vi "svx_Orbit IndexToCheckbox.vi"(4 "All Children Tags":string[](array[string]), 6 "All parents Tags":string[](array[string]), 9 "ColumnIdx":i32, 10 "RowIdx":i32, 11 "Tree ref in":refnum<vi>) -> (3 "Tree ref out":refnum<vi>)   [LabVIEW 2017, in "SVX Orbit.xctl"]
uses:
  <vilib>/addons/_XControls/Orbit Plot/SVX Orbit.xctl
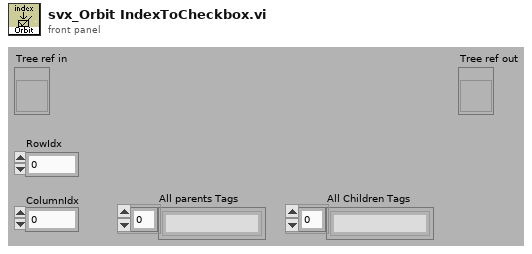
[diagram p1: front panel]
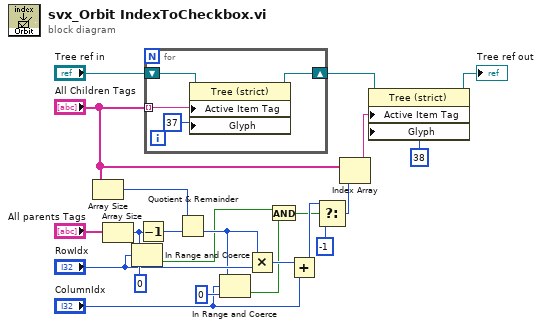
[diagram p0: block diagram]
diagram:
  n1 = Array Size(array="All Children Tags") -> (size(s)=w13:i32)
  n2 = Array Size(array="All parents Tags") -> (size(s)=w11:i32)
  n3 = In Range and Coerce(upper limit=w11, x="RowIdx", lower limit=0) -> (In Range?=w6:bool)  [unwired: 1 out]
  n4 = Decrement(x=w11) -> (x-1=w15:i32)
  n5 = for {
    tunnel: "All Children Tags" -> [w25] mode=indexing
    shift-right: [w23] -> w20
    shift-left: "Tree ref in" -> [w26]
    n6 = property class="Tree (strict)"(reference=w26, "Active Item Tag"=w25, "Glyph"=37 ("Active Item:Symbol Index")) -> (reference out=w23:refnum<vi>)  [unwired: 1 in, 1 out]
  }
  n7 = Quotient & Remainder(x=w13, y=w15) -> (floor(x/y)=w7:i32)  [unwired: 1 out]
  n8 = In Range and Coerce(upper limit=w7, x="ColumnIdx", lower limit=0) -> (In Range?=w5:bool)  [unwired: 1 out]
  n9 = Multiply(x=w7, y="RowIdx") -> (x*y=w21:i32)
  n10 = And(x=w6, y=w5) -> (x .and. y?=w1:bool)
  n11 = Add(x=w21, y="ColumnIdx") -> (x+y=w2:i32)
  n12 = Select(t=w2, s=w1, f=-1 ("t")) -> (s? t:f=w3:i32)
  n13 = Index Array(array="All Children Tags", index=w3) -> (element=w19:string)
  n14 = property class="Tree (strict)"(reference=w20, "Active Item Tag"=w19, "Glyph"=38 ("Active Item:Symbol Index")) -> (reference out=→"Tree ref out":refnum<vi>)  [unwired: 1 in, 1 out]
